vi "Read Register (Core).vi"(0 "SLSC Interface in":refnum<class "SLSC Interface.lvclass">, 1 "type":enum16{"U8", "U16", "U32", "U64"}(ring), 5 "device":refnum<k21>="$DefaultDevices", 7 "register address":u32 format="%.0x", 11 "error in (no error)":errorcluster) -> (4 "SLSC Interface out":refnum<class "SLSC Interface.lvclass">, 6 "device out":refnum<k21>, 8 "next register address":u32 format="%.0x", 10 "data out":u64 format="%.0x", 15 "error out":errorcluster)   [LabVIEW 2015, in "SLSC Interfaces.lvlib" / "SLSC Interface.lvclass"]
uses:
  SLSC Interface.lvclass
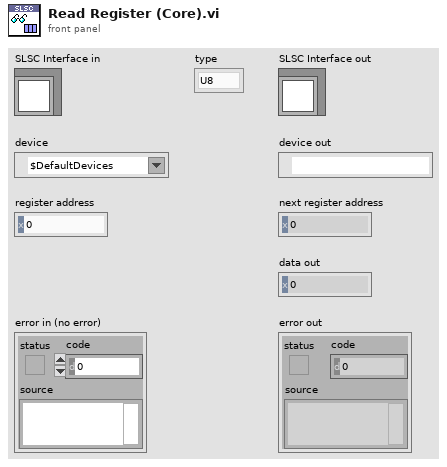
[diagram p1: front panel]
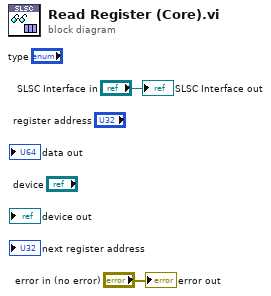
[diagram p0: block diagram]
diagram:
  "error out" <- "error in (no error)"
  "SLSC Interface out" <- "SLSC Interface in"
